vi "Gradient Read Array.vi"(8 "error in":errorcluster, 11 "Current Gradient in":refnum<class "Current Gradient.lvclass">) -> (0 "error out":errorcluster, 1 "Changed or First Call?":bool, 2 "Current SP":dbl[](array[numeric]), 3 "Current Gradient out":refnum<class "Current Gradient.lvclass">)   [LabVIEW 2023, in "Current Gradient.lvclass"]
uses:
  Current Gradient.lvclass
  Current Gradient.lvclass/Current Gradient.ctl
  Parents/Gradient/Gradient.lvclass
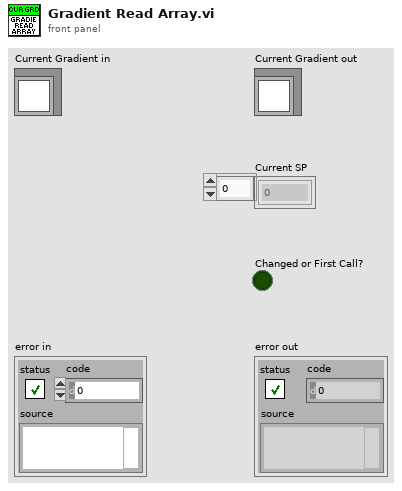
[diagram p1: front panel]
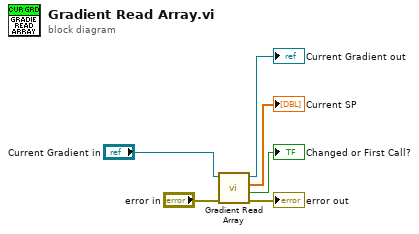
[diagram p0: block diagram]
diagram:
  n1 = call-parent "Gradient Read Array.vi"("error in"="error in", "Gradient in"="Current Gradient in") -> ("error out"=→"error out":errorcluster, "Changed or First Call?"=→"Changed or First Call?":bool, "Current SP"=→"Current SP":dbl[], "Gradient out"=→"Current Gradient out":refnum<class "Current Gradient.lvclass">)  [unwired: 6 in]
